vi "Create New JSON File.vi"(7 "Source Base JSON File":path, 8 "error in":errorcluster, 9 "Slot 2 Module Selection":T1, 10 "Slot 1 Module Selection":T1, 11 "Output Directory":path=path "C:/Users/Tanner Blair/Desktop/SET 2010 Support/output") -> (0 "error out":errorcluster, 3 "path out":path)   [LabVIEW 2017]
uses:
  Slot Module Selection.ctl
  <vilib>/National Instruments/Variant Data Manipulation/Path API/Read Value at Path(String).vi
  <vilib>/National Instruments/Variant Data Manipulation/Path API/Write Value at Path(String).vi
  <vilib>/National Instruments/Variant JSON API/To File (Path).vi
  <vilib>/National Instruments/Variant JSON API/Variant JSON API.lvlib
  <vilib>/National Instruments/Variant Data Manipulation/Variant Data Manipulation.lvlib
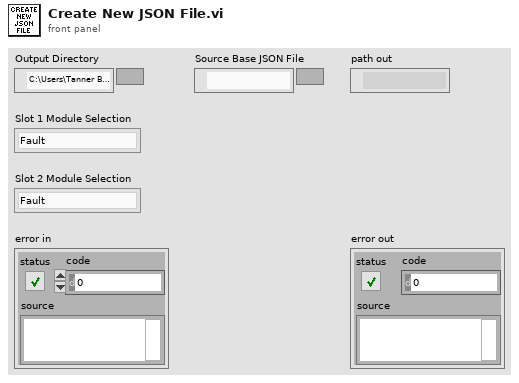
[diagram p1: front panel]
types:
  T1 = typedef "Slot Module Selection.ctl" = enum16{"Fault", "Instrument", "Empty"}
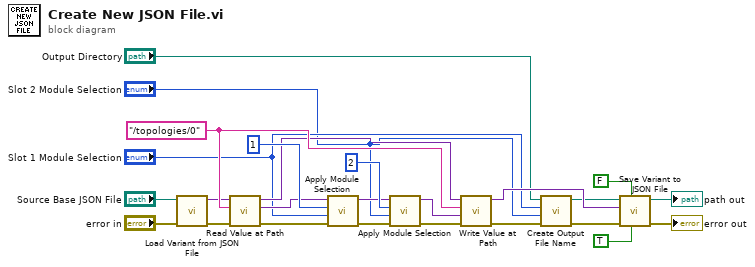
[diagram p0: block diagram]
diagram:
  w10 = "/topologies/0" ("Path String")
  n1 = call <vilib>:"Load Variant from JSON File.vi"("error in"="error in", "file path"="Source Base JSON File") -> ("error out"=w11:errorcluster, "Variant out"=w8:variant)  [unwired: 8 in]
  n2 = call-poly <vilib>:"Read Value at Path.vi"("error in (no error)"=w11, "Path String"=w10, "Variant in"=w8) -> ("error out"=w14:errorcluster, "Element out"=w15:variant, "Variant out"=w9:variant)  [unwired: 6 in]
  n3 = call "Apply Module Selection.vi"("error in (no error)"=w14, "Module Type"="Slot 1 Module Selection", "Slot # in"=1 ("Slot #"), "Base Topology Variant in"=w15) -> ("error out"=w12:errorcluster, "Base Topology Variant out"=w18:variant)  [unwired: 6 in]
  n4 = call "Apply Module Selection.vi"("error in (no error)"=w12, "Module Type"="Slot 2 Module Selection", "Slot # in"=2, "Base Topology Variant in"=w18) -> ("error out"=w17:errorcluster, "Base Topology Variant out"=w19:variant)  [unwired: 6 in]
  n5 = call-poly <vilib>:"Write Value at Path.vi"("error in (no error)"=w17, "Element in"=w19, "Path String"=w10, "Variant in"=w9) -> ("error out"=w2:errorcluster, "Variant out"=w21:variant)  [unwired: 6 in]
  n6 = call "Create Output File Name.vi"("error in (no error)"=w2, "Slot 2 Module Selection"="Slot 2 Module Selection", "Slot 1 Module Selection"="Slot 1 Module Selection", "Output Directory"="Output Directory") -> ("error out"=w1:errorcluster, "output file name"=w3:path)  [unwired: 6 in]
  n7 = call-poly <vilib>:"Save Variant to JSON File.vi"("enable LabVIEW extensions? (T)"=TRUE, "Pretty Print?"=FALSE, "error in (no error)"=w1, "Variant in"=w21, "path in"=w3) -> ("error out"=→"error out":errorcluster, "path out"=→"path out":path)  [unwired: 5 in]
